vi "Configure Detector List.vi"(8 "error in (no error)":errorcluster, 10 "Detector List":i32[](array[ring])=[0, 0, 0] items=["LAVG", "VAVG", "RMS", "Negative", "Positive", "Sample", "Peak-AVER", "Peak-RMS", "DualAvg"], 11 "VISA resource name":refnum<visa-resource-name>) -> (0 "error out":errorcluster, 3 "VISA resource name out":refnum<visa-resource-name>)   [LabVIEW 2014, in "Agilent MXA Series.lvlib"]
doc: "Cofigures the Detector type under List Sweep measurement type."
uses:
  Agilent MXA Series.lvlib
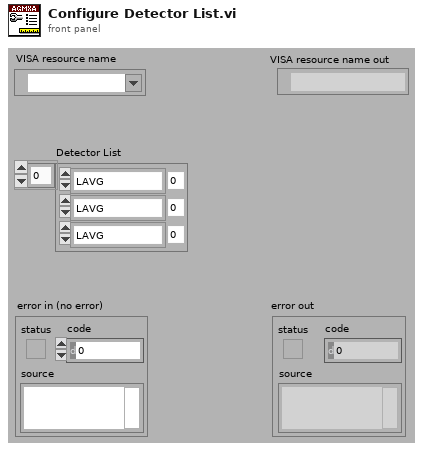
[diagram p1: front panel]
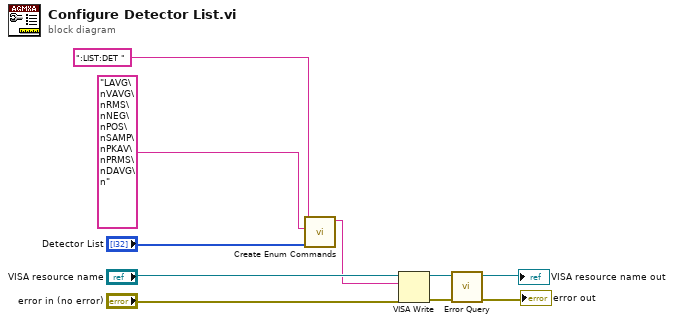
[diagram p0: block diagram]
diagram:
  n1 = call "Create Enum Commands.vi"("Enum Values"="Detector List", "Multi-line Text"="LAVG\nVAVG\nRMS\nNEG\nPOS\nSAMP\nPKAV\nPRMS\nDAVG\n" ("multi-line string"), "Commands"=":LIST:DET ") -> ("Result"=w1:string)  [unwired: 8 in]
  n2 = VISA Write(VISA resource name="VISA resource name", write buffer=w1, error in (no error)="error in (no error)") -> (VISA resource name out=w7:refnum<visa-resource-name>, error out=w8:errorcluster)  [unwired: 1 out]
  n3 = call "Error Query.vi"("error in (no error)"=w8, "VISA resource name"=w7) -> ("error out"=→"error out":errorcluster, "VISA resource name out"=→"VISA resource name out":refnum<visa-resource-name>)  [unwired: 6 in, 2 out]
